vi "MainScreen.vi"() -> ()   [LabVIEW 2015]
panel:
  out "时间显示":timestamp format="%<%X    %x   %A>T"
  out "公司信息":string="名称：上海仪杰自动化设备有限公司  地址：上海浦东新区彭镇银河路  电话：021-58244212                                                                    程序版本：V1.0"
  out "测试结果":string
  in  "手动状态":bool
  in  "自动状态":bool
  out "状态信息":string
  in  "功能选项卡":enum32{"产品参数", "相机参数", "系统状态", "手动界面"}(tab)
  out "产品图像":T1(plugin-control)
  out "标准模板":T1(plugin-control)
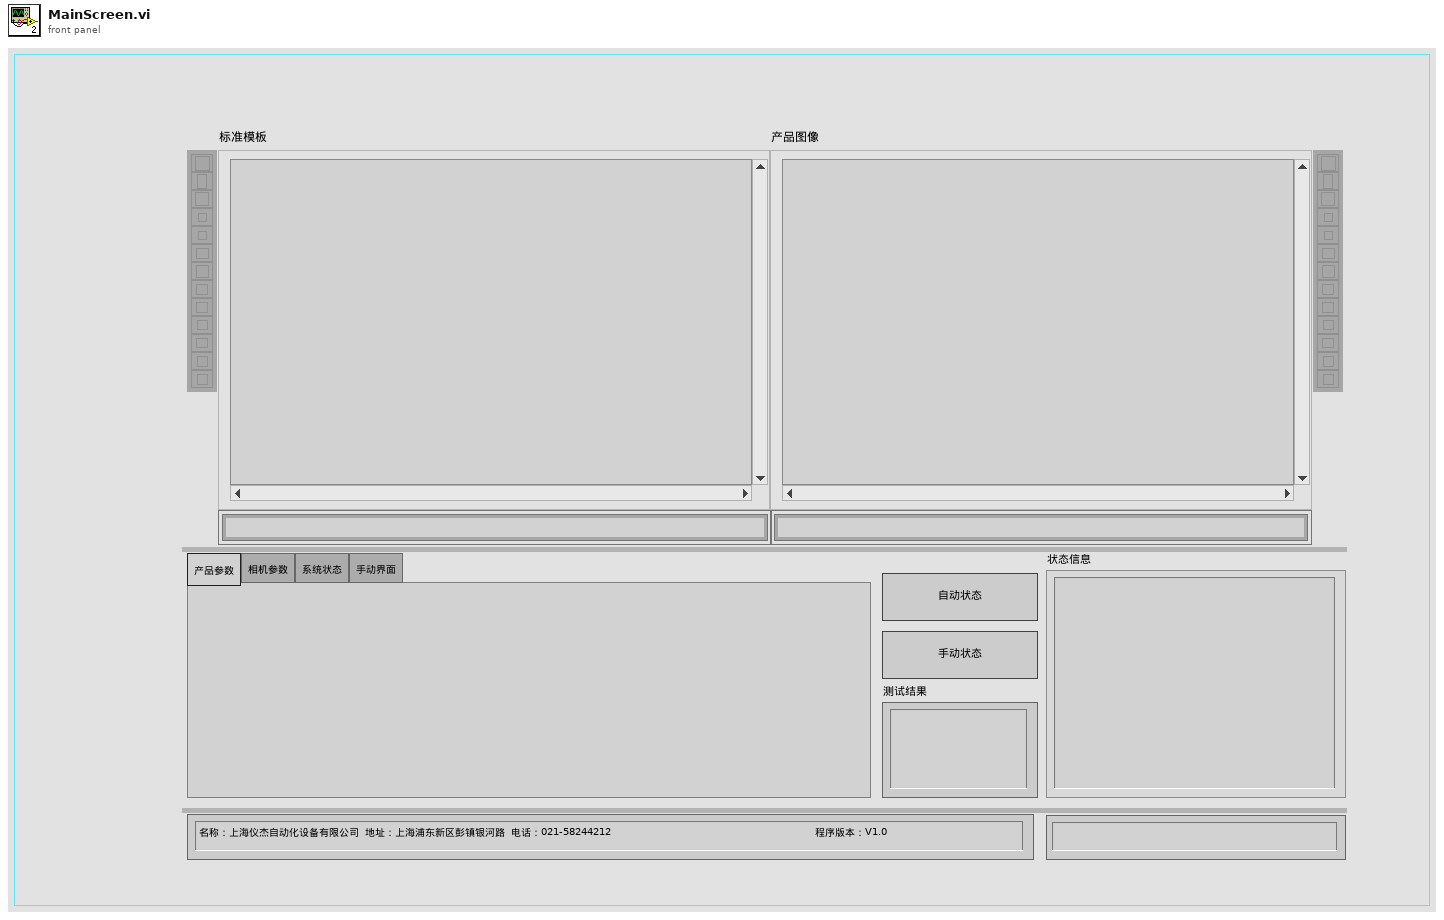
[diagram p1: front panel]
types:
  T1 = typedef "IMAQ Image.ctl" = refnum<image>
  T2 = typedef "控件_逻辑过程.ctl" = enum16{"初始化", "等待执行", "处理结果", "存储数据", "错误处理", "关闭程序", ""}
  T3 = cluster{"逻辑过程":T2, "菜单命令":string, "功能选项卡":enum32{"产品参数", "相机参数", "系统状态", "手动界面"}, "按钮事件":cluster{"名称":string, "值":bool}}
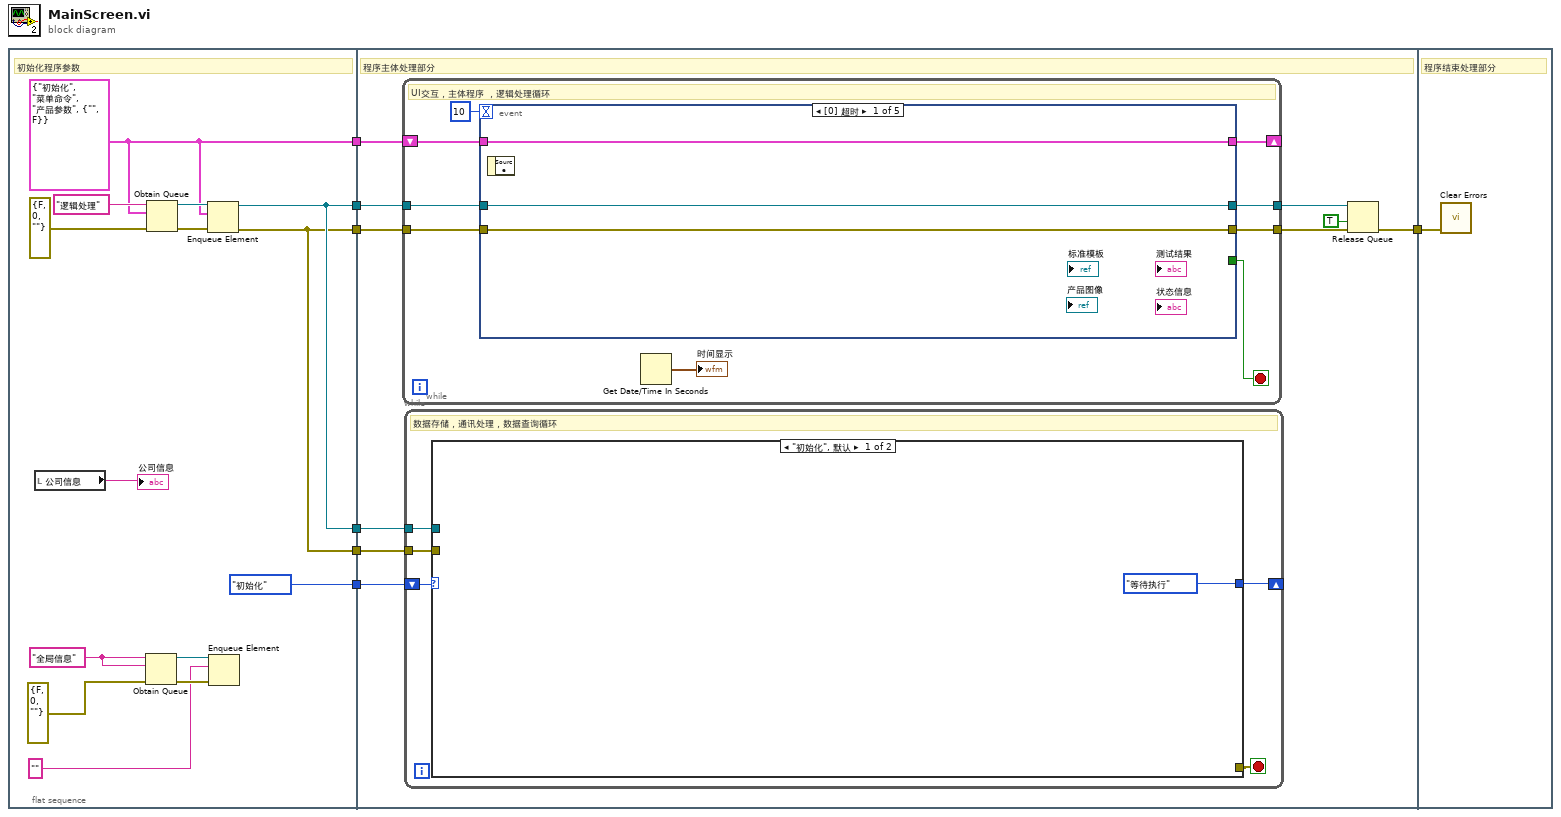
[diagram p0: block diagram]
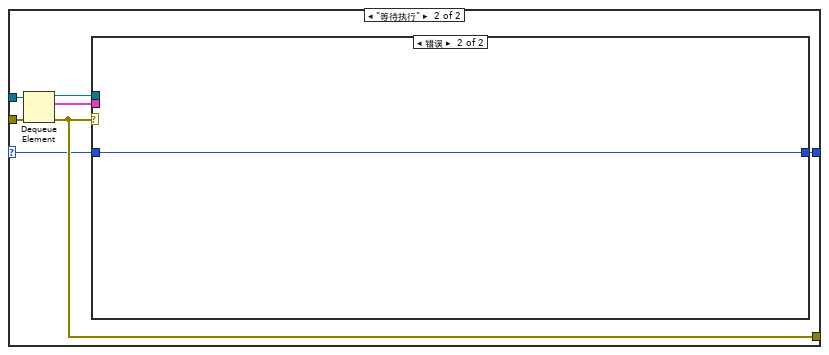
[diagram p2: hidden frame]
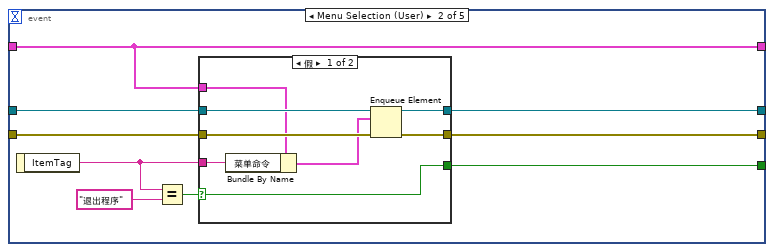
[diagram p4: hidden frame]
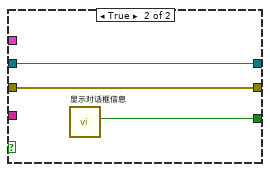
[diagram p5: hidden frame]
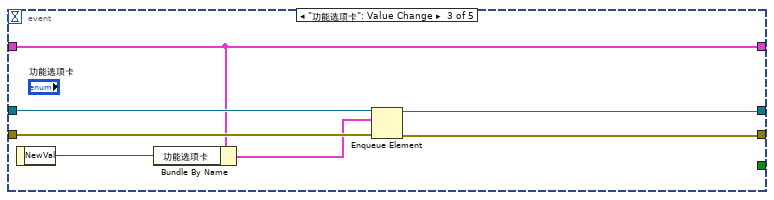
[diagram p6: hidden frame]
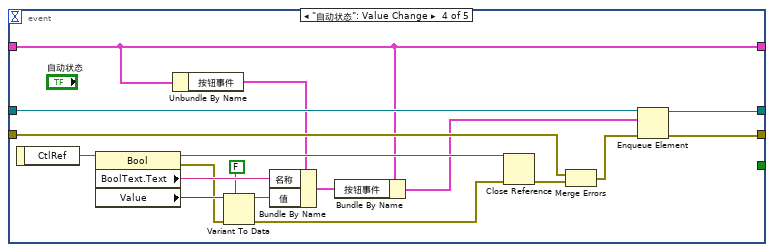
[diagram p7: hidden frame]
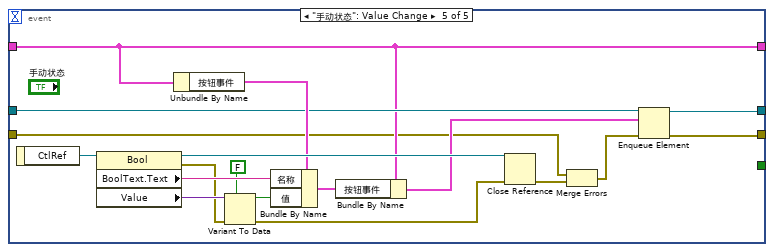
[diagram p8: hidden frame]
diagram:
  n1 = flat-sequence {
    tunnel: [w16] -> w7
    tunnel: [w17] -> w6
    tunnel: [w17] -> w4
    tunnel: [w16] -> w3
    tunnel: [w10] -> w2
    tunnel: [控件_逻辑过程."初始化" ("逻辑过程")] -> w1
    tunnel: w7 -> [w31]
    tunnel: w6 -> [w30]
    tunnel: [w24] -> w5
    tunnel: w4 -> [w29]
    tunnel: w3 -> [w28]
    tunnel: w2 -> [w23]
    tunnel: w1 -> [w22]
    tunnel: w5 -> [w122]
    frame #0 {
      w10 = T3 {"逻辑过程"=enum."初始化", "菜单命令"="菜单命令", "功能选项卡"=enum."产品参数", "按钮事件"={"名称"="", "值"=FALSE}}
      w13 = "全局信息"
      # "初始化程序参数"
      n2 = local read "公司信息"() -> (→"公司信息":string)
      n3 = Obtain Queue(name (unnamed)=w13, element data type=w13, error in (no error)=errorcluster {"status"=FALSE, "code"=0, "source"=""} ("错误常量")) -> (queue out=w14:refnum<queue>, error out=w15:errorcluster)  [unwired: 2 in, 1 out]
      n4 = Obtain Queue(name (unnamed)="逻辑处理", element data type=w10, error in (no error)=errorcluster {"status"=FALSE, "code"=0, "source"=""} ("错误常量")) -> (queue out=w20:refnum<queue>, error out=w19:errorcluster)  [unwired: 2 in, 1 out]
      n5 = Enqueue Element(queue=w20, element=w10, error in (no error)=w19) -> (queue out=w17:refnum<queue>, error out=w16:errorcluster)  [unwired: 1 in, 1 out]
      n6 = Enqueue Element(queue=w14, element="", error in (no error)=w15) -> ()  [unwired: 1 in, 3 out]
    }
    frame #1 {
      # "程序主体处理部分"
      n7 = while {
        tunnel: w30 -> [w55]
        tunnel: [w53] -> w26
        tunnel: w31 -> [w54]
        tunnel: [w52] -> w25
        shift-right: [w49] -> _
        shift-left: w23 -> [w50]
        stop <- w51 stop-if-true
        # "UI交互，主体程序 ，逻辑处理循环"
        n8 = event shown="[0] 超时" {
          selector: _ -> [_ _ _ _ _]
          dyn-events: _ -> [_ _ _ _ _]
          timeout: 10 -> [_ _ _ _ _]
          tunnel: w55 -> [w57 w67 w84 w103 w109]
          tunnel: w54 -> [w56 w65 w83 w90 w107]
          tunnel: [w57 w66 w82 w102 w106] -> w53
          tunnel: [w56 w64 w81 w101 w105] -> w52
          tunnel: [_ w59 _ _ _] -> w51
          tunnel: w50 -> [w58 w63 w80 w87 w108]
          tunnel: [w58 w63 w80 w87 w108] -> w49
          event Timeout {
            n9 = event-data() -> ()  [unwired: 1 in, 1 out]
          }
          event Menu Selection (User) {
            n10 = event-data() -> ("ItemTag"=w62:string)  [unwired: 1 in]
            n11 = Equal?(x=w62, y="退出程序") -> (x = y?=w61:bool)
            n12 = case shown="假" w61 {
              selector: w61 -> [w68 _]
              tunnel: w67 -> [w75 w78]
              tunnel: [w74 w78] -> w66
              tunnel: w65 -> [w73 w77]
              tunnel: [w72 w77] -> w64
              tunnel: w63 -> [w71 _]
              tunnel: w62 -> [w69 _]
              tunnel: [w68 w76] -> w59
              frame False {
                n13 = Bundle By Name(cluster=w71, "菜单命令"=w69) -> (w70:T3)
                n14 = Enqueue Element(queue=w75, element=w70, error in (no error)=w73) -> (queue out=w74:refnum<queue>, error out=w72:errorcluster)  [unwired: 1 in, 1 out]
              }
              frame True {
                n15 = call "显示对话框信息"() -> ("确定"=w76:bool)  [unwired: 10 in, 1 out]
              }
            }
          }
          event "功能选项卡": Value Change {
            n16 = event-data() -> ("NewVal"=w85:enum32{"产品参数", "相机参数", "系统状态", "手动界面"})  [unwired: 1 in]
            n17 = Bundle By Name(cluster=w80, "功能选项卡"=w85) -> (w79:T3)
            n18 = Enqueue Element(queue=w84, element=w79, error in (no error)=w83) -> (queue out=w82:refnum<queue>, error out=w81:errorcluster)  [unwired: 1 in, 1 out]
          }
          event "自动状态": Value Change {
            n19 = event-data() -> ("CtlRef"=w99:refnum<vi>)  [unwired: 1 in]
            n20 = property class="Bool"(reference=w99) -> (reference out=w94:refnum<vi>, error out=w93:errorcluster, "BoolText.Text"=w98:string, "Value"=w97:variant)  [unwired: 1 in]
            n21 = Unbundle By Name(w87) -> ("按钮事件"=w88:cluster{"名称":string, "值":bool})
            n22 = Variant To Data(error in=w93, type=FALSE, Variant=w97) -> (data=w95:bool, error out=w92:errorcluster)
            n23 = Bundle By Name(cluster=w88, "名称"=w98, "值"=w95) -> (w100:cluster{"名称":string, "值":bool})
            n24 = Bundle By Name(cluster=w87, "按钮事件"=w100) -> (w86:T3)
            n25 = Close Reference(reference=w94, error in (no error)=w92) -> (error out=w91:errorcluster)
            n26 = Merge Errors(w90, w91) -> (w89:errorcluster)
            n27 = Enqueue Element(queue=w103, element=w86, error in (no error)=w89) -> (queue out=w102:refnum<queue>, error out=w101:errorcluster)  [unwired: 1 in, 1 out]
          }
          event "手动状态": Value Change {
            n28 = event-data() -> ("CtlRef"=w104:refnum<vi>)  [unwired: 1 in]
            n29 = property class="Bool"(reference=w104) -> (reference out=w116:refnum<vi>, error out=w115:errorcluster, "BoolText.Text"=w120:string, "Value"=w119:variant)  [unwired: 1 in]
            n30 = Unbundle By Name(w108) -> ("按钮事件"=w111:cluster{"名称":string, "值":bool})
            n31 = Variant To Data(error in=w115, type=FALSE, Variant=w119) -> (data=w117:bool, error out=w114:errorcluster)
            n32 = Bundle By Name(cluster=w111, "名称"=w120, "值"=w117) -> (w121:cluster{"名称":string, "值":bool})
            n33 = Bundle By Name(cluster=w108, "按钮事件"=w121) -> (w110:T3)
            n34 = Close Reference(reference=w116, error in (no error)=w114) -> (error out=w113:errorcluster)
            n35 = Merge Errors(w107, w113) -> (w112:errorcluster)
            n36 = Enqueue Element(queue=w109, element=w110, error in (no error)=w112) -> (queue out=w106:refnum<queue>, error out=w105:errorcluster)  [unwired: 1 in, 1 out]
          }
        }
        n37 = Get Date/Time In Seconds() -> (seconds since 1Jan1904=→"时间显示":timestamp)
      }
      n38 = while {
        tunnel: w29 -> [w36]
        tunnel: w28 -> [w35]
        shift-right: [w32] -> _
        shift-left: w22 -> [w33]
        stop <- w34 stop-if-true
        # "数据存储，通讯处理，数据查询循环"
        n39 = case shown="\"初始化\", 默认" w33 {
          selector: w33 -> [_ w39]
          tunnel: w36 -> [_ w44]
          tunnel: w35 -> [_ w43]
          tunnel: [_ w40] -> w34
          tunnel: [控件_逻辑过程."等待执行" ("逻辑过程") w38] -> w32
          frame "初始化", Default {
          }
          frame "等待执行" {
            n40 = Dequeue Element(queue=w44, error in (no error)=w43) -> (queue out=w42:refnum<queue>, element=w41:T3, error out=w40:errorcluster)  [unwired: 1 in, 1 out]
            n41 = case shown="错误" w40 {
              tunnel: w42 -> [_ _]
              tunnel: w41 -> [_ _]
              tunnel: w39 -> [w45 w46]
              tunnel: [w45 w46] -> w38
              frame No Error {
              }
              frame Error {
              }
            }
          }
        }
      }
      n42 = Release Queue(queue=w26, force destroy? (F)=TRUE ("强制销毁？(F)"), error in (no error)=w25) -> (error out=w24:errorcluster)  [unwired: 2 out]
    }
    frame #2 {
      # "程序结束处理部分"
      n43 = call <vilib>:"Clear Errors.vi"("error in (no error)"=w122) -> ()  [unwired: 5 in, 2 out]
    }
  }
